vi "ReadWaveform.vi"(7 "Poll Time (ms)":u32=10, 8 "error in":errorcluster, 9 "Timeout (s)":dbl=5.0, 10 "Samps Read per Chan":i32, 11 "Task in":refnum<class "WaveformTask.lvclass">) -> (0 "error out":errorcluster, 1 "Samples Remaining":u32, 2 "Waveforms":waveform(sgl)[](array[waveform]), 3 "Task out":refnum<class "WaveformTask.lvclass">)   [LabVIEW 2015, in "WaveformTask.lvclass"]
uses:
  WaveformTask.lvclass
  WaveformTask.lvclass/WaveformTask.ctl
  <vilib>/NI/cRIO Wfm/ErrorSelector.ctl
  <vilib>/rvi/errors/niLvFpgaAdjustHostInterfaceError.vi
  <vilib>/Utility/error.llb/Error Cluster From Error Code.vi
  DataFIFOs.ctl
  <vilib>/rvi/interface/nirviMethod/nirviMethod.xnode
  <vilib>/NI/cRIO Wfm/cRIO Wfm.lvlib
  <vilib>/FPGAPlugInAG/Dynamic/niLvFpga_ReadFifo_Dynamic.vi
  <vilib>/rvi/errors/niLvFpgaMergeErrorWithErrorCode.vi
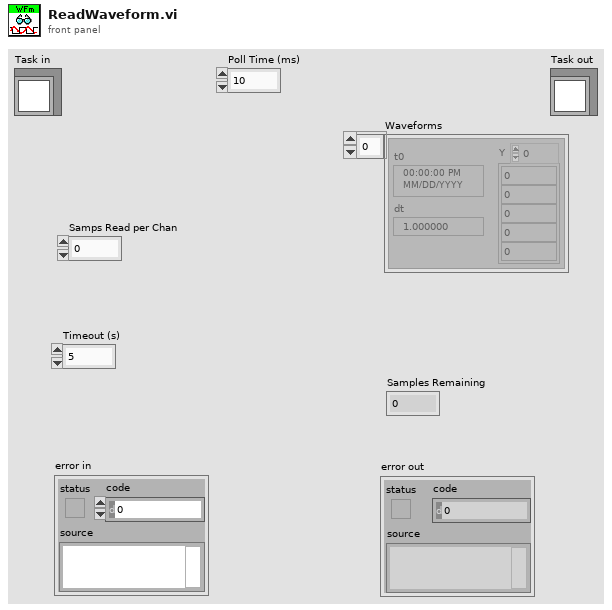
[diagram p1: front panel]
types:
  T1 = typedef "WaveformTask.lvclass/DataFIFOs.ctl" = refnum<k20>
  T2 = typedef "cRIO Wfm.lvlib/ErrorSelector.ctl" = enum16{"Read Timeout", "Module Underflow", "DMA Overflow", "Chan Count", "Run Timeout", "Start Timeout", "Stop Timeout"}
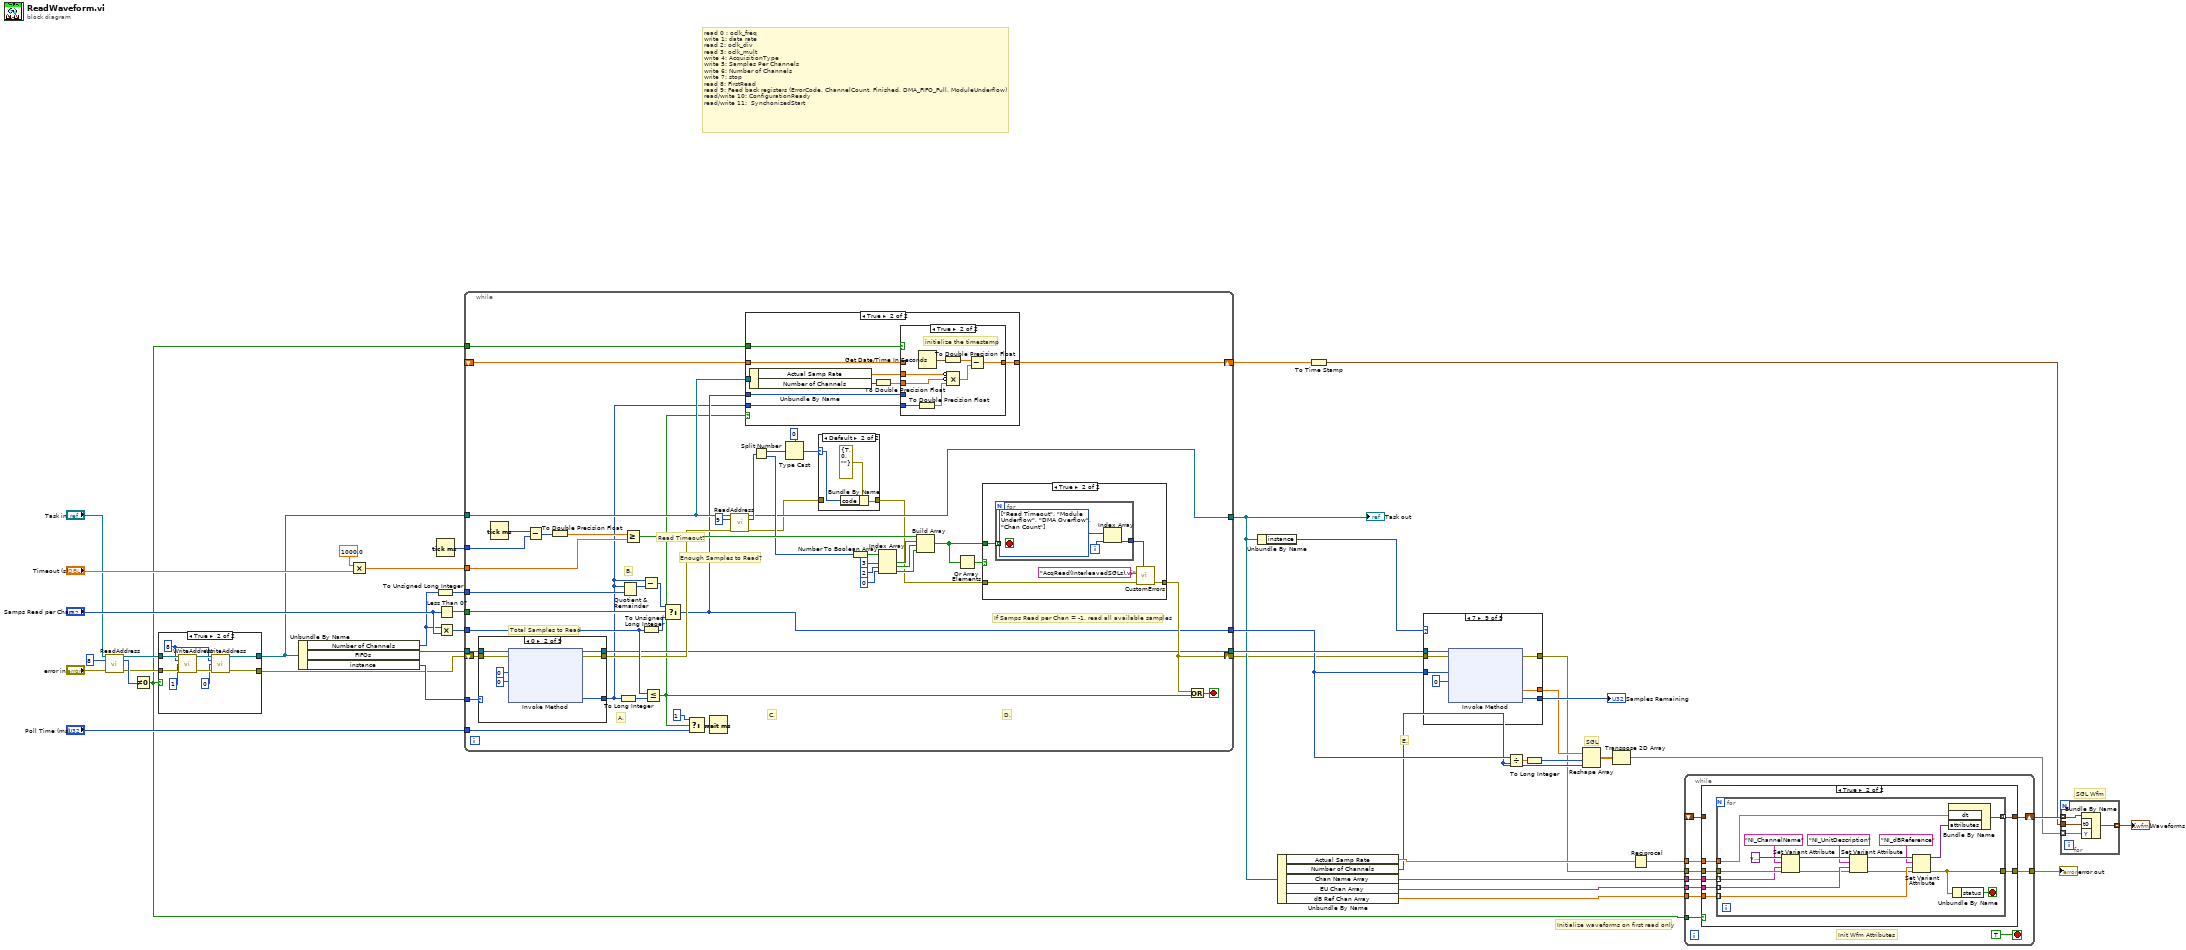
[diagram p0: block diagram]
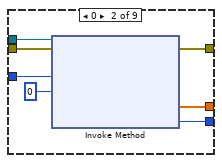
[diagram p5: hidden frame]
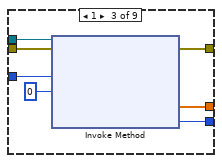
[diagram p6: hidden frame]
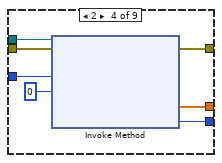
[diagram p7: hidden frame]
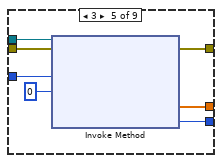
[diagram p8: hidden frame]
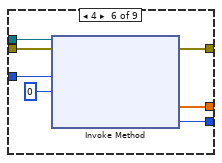
[diagram p9: hidden frame]
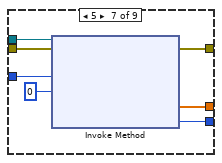
[diagram p10: hidden frame]
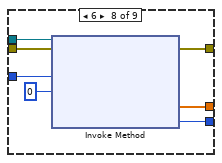
[diagram p11: hidden frame]
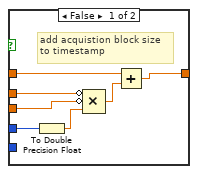
[diagram p13: hidden frame]
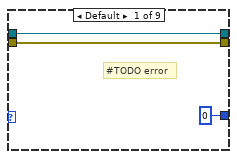
[diagram p15: hidden frame]
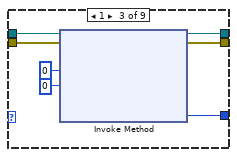
[diagram p16: hidden frame]
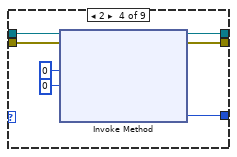
[diagram p17: hidden frame]
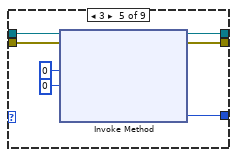
[diagram p18: hidden frame]
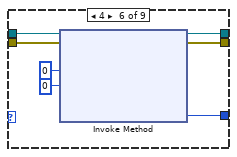
[diagram p19: hidden frame]
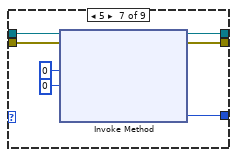
[diagram p20: hidden frame]
diagram:
  # "Initialize waveforms on first read only"
  # "SGL Wfm"
  # "SGL"
  # "read 0 : oclk_freq\nwrite 1: data rate\nread 2: oclk_div\nread 3: oclk_mult\nwrite 4: AcquisitionType\nwrite 5: Samples Per Channels\nwrite 6: Number of Channels\nwrite 7: stop\nread 8: FirstRead\nread 9: Feed back registers (ErrorCode, ChannelCount, Finished, DMA_FIFO_Full, ModuleUnderflow)\nread/write 10: ConfigurationReady\nread/write 11:  SynchonizedStart"
  # "E."
  n1 = call "ReadAddress.vi"("Task in"="Task in", "address"=u64 8, "error in (no error)"="error in") -> ("Task out"=w6:refnum<class "WaveformTask.lvclass">, "data"=w7:u64, "error out"=w5:errorcluster)  [unwired: 10 in]
  n2 = Not Equal To 0?(x=w7) -> (x != 0?=w2:bool)
  n3 = case shown="True" w2 {
    tunnel: w6 -> [w46 w55]
    tunnel: w5 -> [w45 w54]
    tunnel: [w46 w48] -> w4
    tunnel: [w45 w47] -> w3
    frame False {
    }
    frame True {
      w51 = u64 8 ("address")
      n4 = call "WriteAddress.vi"("Task in"=w55, "address"=w51, "data"=u64 1, "error in (no error)"=w54) -> ("Task out"=w53:refnum<class "WaveformTask.lvclass">, "error out"=w52:errorcluster)  [unwired: 10 in]
      n5 = call "WriteAddress.vi"("Task in"=w53, "address"=w51, "data"=u64 0, "error in (no error)"=w52) -> ("Task out"=w48:refnum<class "WaveformTask.lvclass">, "error out"=w47:errorcluster)  [unwired: 10 in]
    }
  }
  n6 = Unbundle By Name(w4) -> ("Number of Channels"=w32:i32, "FIFOs"=w33:T1, "instance"=w31:u8)
  n7 = Multiply(x=1000.0 ("y"), y="Timeout (s)") -> (x*y=w42:dbl)
  n8 = To Unsigned Long Integer(number=w32) -> (unsigned 32bit integer=w38:u32)
  n9 = Tick Count (ms)() -> (millisecond timer value=w44:u32)
  n10 = Less Than 0?(x="Samps Read per Chan") -> (x < 0?=w40:bool)
  n11 = Multiply(x=w32, y="Samps Read per Chan") -> (x*y=w39:i32)
  n12 = while {
    tunnel: [w68] -> w41
    tunnel: w33 -> [w98]
    tunnel: w44 -> [w100]
    tunnel: w42 -> [w99]
    tunnel: "Poll Time (ms)" -> [w93]
    tunnel: [w58] -> w25
    tunnel: w39 -> [w88]
    tunnel: w40 -> [w89]
    tunnel: w38 -> [w90]
    shift-right: [w82] -> w16
    shift-left: w3 -> [w97]
    tunnel: w4 -> [w62]
    tunnel: [w67] -> w18
    tunnel: w31 -> [w66]
    tunnel: w2 -> [w61]
    shift-right: [w60] -> w1
    shift-left: _ -> [w59]
    stop <- w103 stop-if-true
    # "A."
    # "D."
    # "C."
    # "B."
    # "If Samps Read per Chan = -1, read all available samples"
    # "Read Timeout?"
    # "Total Samples to Read"
    # "Enough Samples to Read?"
    n13 = case shown="0" w66 {
      tunnel: w98 -> [w135 w142 w149 w156 w163 w170 w177 w184 w191]
      tunnel: w97 -> [w134 w141 w148 w155 w162 w169 w176 w183 w190]
      tunnel: [u32 0 ("Elements Remaining") w138 w145 w152 w159 w166 w173 w180 w187] -> w56
      tunnel: [w134 w137 w144 w151 w158 w165 w172 w179 w186] -> w75
      tunnel: [w135 w136 w143 w150 w157 w164 w171 w178 w185] -> w68
      frame Default {
        # "#TODO error"
      }
      frame 0 {
        n14 = xnode "Invoke Method"("FPGA VI Reference In"=w142, "error in"=w141, "Number of Elements"=u32 0, "Timeout (ms)"=0) -> ("FPGA VI Reference Out"=w136:T1, "error out"=w137:errorcluster, "Elements Remaining"=w138:u32)  [unwired: 1 out]
      }
      frame 1 {
        n15 = xnode "Invoke Method"("FPGA VI Reference In"=w149, "error in"=w148, "Number of Elements"=u32 0, "Timeout (ms)"=0) -> ("FPGA VI Reference Out"=w143:T1, "error out"=w144:errorcluster, "Elements Remaining"=w145:u32)  [unwired: 1 out]
      }
      frame 2 {
        n16 = xnode "Invoke Method"("FPGA VI Reference In"=w156, "error in"=w155, "Number of Elements"=u32 0, "Timeout (ms)"=0) -> ("FPGA VI Reference Out"=w150:T1, "error out"=w151:errorcluster, "Elements Remaining"=w152:u32)  [unwired: 1 out]
      }
      frame 3 {
        n17 = xnode "Invoke Method"("FPGA VI Reference In"=w163, "error in"=w162, "Number of Elements"=u32 0, "Timeout (ms)"=0) -> ("FPGA VI Reference Out"=w157:T1, "error out"=w158:errorcluster, "Elements Remaining"=w159:u32)  [unwired: 1 out]
      }
      frame 4 {
        n18 = xnode "Invoke Method"("FPGA VI Reference In"=w170, "error in"=w169, "Number of Elements"=u32 0, "Timeout (ms)"=0) -> ("FPGA VI Reference Out"=w164:T1, "error out"=w165:errorcluster, "Elements Remaining"=w166:u32)  [unwired: 1 out]
      }
      frame 5 {
        n19 = xnode "Invoke Method"("FPGA VI Reference In"=w177, "error in"=w176, "Number of Elements"=u32 0, "Timeout (ms)"=0) -> ("FPGA VI Reference Out"=w171:T1, "error out"=w172:errorcluster, "Elements Remaining"=w173:u32)  [unwired: 1 out]
      }
      frame 6 {
        n20 = xnode "Invoke Method"("FPGA VI Reference In"=w184, "error in"=w183, "Number of Elements"=u32 0, "Timeout (ms)"=0) -> ("FPGA VI Reference Out"=w178:T1, "error out"=w179:errorcluster, "Elements Remaining"=w180:u32)  [unwired: 1 out]
      }
      frame 7 {
        n21 = xnode "Invoke Method"("FPGA VI Reference In"=w191, "error in"=w190, "Number of Elements"=u32 0, "Timeout (ms)"=0) -> ("FPGA VI Reference Out"=w185:T1, "error out"=w186:errorcluster, "Elements Remaining"=w187:u32)  [unwired: 1 out]
      }
    }
    n22 = Tick Count (ms)() -> (millisecond timer value=w96:u32)
    n23 = Subtract(x=w96, y=w100) -> (x-y=w102:u32)
    n24 = To Double Precision Float(number=w102) -> (double precision float=w101:dbl)
    n25 = To Long Integer(number=w56) -> (32bit integer=w91:i32)
    n26 = Quotient & Remainder(x=w56, y=w90) -> (x-y*floor(x/y)=w86:u32)  [unwired: 1 out]
    n27 = Greater Or Equal?(x=w101, y=w99) -> (x >= y?=w95:bool)
    n28 = Subtract(x=w56, y=w86) -> (x-y=w85:u32)
    n29 = To Unsigned Long Integer(number=w88) -> (unsigned 32bit integer=w87:u32)
    n30 = Less Or Equal?(x=w88, y=w91) -> (x <= y?=w57:bool)
    n31 = Select(t=w85, s=w89, f=w87) -> (s? t:f=w58:u32)
    n32 = Select(t=u32 1, s=w57, f=w93) -> (s? t:f=w94:u32)
    n33 = Wait (ms)(milliseconds to wait=w94) -> ()  [unwired: 1 out]
    n34 = call "ReadAddress.vi"("Task in"=w62, "address"=u64 9, "error in (no error)"=w75) -> ("Task out"=w67:refnum<class "WaveformTask.lvclass">, "data"=w80:u64, "error out"=w64:errorcluster)  [unwired: 10 in]
    n35 = case shown="True" w57 {
      tunnel: w59 -> [w104 w113]
      tunnel: w61 -> [_ w112]
      tunnel: w62 -> [_ w110]
      tunnel: w56 -> [_ w109]
      tunnel: [w104 w108] -> w60
      tunnel: w58 -> [_ w107]
      frame False {
      }
      frame True {
        n36 = Unbundle By Name(w110) -> ("Actual Samp Rate"=w111:dbl, "Number of Channels"=w106:i32)
        n37 = To Double Precision Float(number=w106) -> (double precision float=w105:dbl)
        n38 = case shown="True" w112 {
          tunnel: w111 -> [w118 w128]
          tunnel: w113 -> [w119 _]
          tunnel: w107 -> [w115 _]
          tunnel: w105 -> [w116 w127]
          tunnel: w109 -> [_ w122]
          tunnel: [w120 w124] -> w108
          frame False {
            # "add acquistion block size\nto timestamp"
            n39 = To Double Precision Float(number=w115) -> (double precision float=w114:dbl)
            n40 = Compound Arithmetic op=MULTIPLY(invert w118, invert w116, w114) -> (w117:dbl)
            n41 = Add(x=w119, y=w117) -> (x+y=w120:dbl)
          }
          frame True {
            # "initialize the timestamp"
            n42 = To Double Precision Float(number=w122) -> (double precision float=w121:dbl)
            n43 = Get Date/Time In Seconds() -> (seconds since 1Jan1904=w126:timestamp)
            n44 = To Double Precision Float(number=w126) -> (double precision float=w123:dbl)
            n45 = Compound Arithmetic op=MULTIPLY(invert w128, invert w127, w121) -> (w125:dbl)
            n46 = Subtract(x=w123, y=w125) -> (x-y=w124:dbl)
          }
        }
      }
    }
    n47 = Split Number(x=w80) -> (hi(x)=w79:u32, lo(x)=w77:u32)
    n48 = Type Cast(type=0, x=w79) -> (*(type *) &x=w65:i32)
    n49 = case shown="Default" w65 {
      selector: w65 -> [_ w131]
      tunnel: w64 -> [w129 _]
      tunnel: [w129 w130] -> w63
      frame 0 {
      }
      frame Default {
        n50 = Bundle By Name(cluster=errorcluster {"status"=TRUE, "code"=0, "source"=""} ("error out"), "code"=w131) -> (w130:errorcluster)
      }
    }
    n51 = Number To Boolean Array(number=w77) -> (Boolean array=w76:bool[])
    n52 = Index Array(array=w76, index #1=3 ("index"), index #2=2 ("index"), index #3=0 ("index")) -> (element #1=w71:bool, element #2=w70:bool, element #3=w69:bool)
    n53 = Build Array(w95, w71, w70, w69) -> (w83:bool[])
    n54 = Or Array Elements(Boolean array=w83) -> (logical OR=w84:bool)
    n55 = case shown="True" w84 {
      tunnel: [w192 w196] -> w82
      tunnel: w63 -> [w192 w197]
      tunnel: w83 -> [_ w195]
      frame False {
      }
      frame True {
        n56 = for {
          tunnel: w195 -> [w201] mode=indexing
          tunnel: [w198] -> w194
          i -> [w199]
          stop <- w201 stop-if-true
          w200 = T2[] [enum."Read Timeout", enum."Module Underflow", enum."DMA Overflow", enum."Chan Count"] items=["Read Timeout", "Module Underflow", "DMA Overflow", "Chan Count", "Run Timeout", "Start Timeout", "Stop Timeout"]
          n57 = Index Array(array=w200, index=w199) -> (element=w198:T2)
        }
        n58 = call <vilib>:"CustomErrors.vi"("Error Selector"=w194, "error in"=w197, "Calling VI"="AcqRead(InterleavedSGLs).vi") -> ("error out"=w196:errorcluster)  [unwired: 8 in]
      }
    }
    n59 = Or(x=w82, y=w57) -> (x .or. y?=w103:bool)
  }
  "Task out" <- w18
  n60 = Unbundle By Name(w18) -> ("instance"=w30:u8)
  n61 = Unbundle By Name(w18) -> ("Actual Samp Rate"=w24:dbl, "Number of Channels"=w17:i32, "Chan Name Array"=w20:string[], "EU Chan Array"=w21:string[], "dB Ref Chan Array"=w22:dbl[])
  n62 = To Time Stamp(1:w1) -> (0:w12:timestamp)
  n63 = case shown="7" w30 {
    tunnel: [w202 w209 w216 w223 w230 w237 w244 w251 w258] -> w15
    tunnel: w16 -> [w202 w208 w215 w222 w229 w236 w243 w250 w257]
    tunnel: w41 -> [_ w207 w214 w221 w228 w235 w242 w249 w256]
    tunnel: w25 -> [_ w206 w213 w220 w227 w234 w241 w248 w255]
    tunnel: [_ w204 w211 w218 w225 w232 w239 w246 w253] -> w26
    tunnel: [_ w203 w210 w217 w224 w231 w238 w245 w252] -> w34
    frame Default {
      # "#TODO Error"
    }
    frame 0 {
      n64 = xnode "Invoke Method"("FPGA VI Reference In"=w207, "error in"=w208, "Number of Elements"=w206, "Timeout (ms)"=0) -> ("error out"=w209:errorcluster, "Data"=w204:sgl[], "Elements Remaining"=w203:u32)  [unwired: 1 out]
    }
    frame 1 {
      n65 = xnode "Invoke Method"("FPGA VI Reference In"=w214, "error in"=w215, "Number of Elements"=w213, "Timeout (ms)"=0) -> ("error out"=w216:errorcluster, "Data"=w211:sgl[], "Elements Remaining"=w210:u32)  [unwired: 1 out]
    }
    frame 2 {
      n66 = xnode "Invoke Method"("FPGA VI Reference In"=w221, "error in"=w222, "Number of Elements"=w220, "Timeout (ms)"=0) -> ("error out"=w223:errorcluster, "Data"=w218:sgl[], "Elements Remaining"=w217:u32)  [unwired: 1 out]
    }
    frame 3 {
      n67 = xnode "Invoke Method"("FPGA VI Reference In"=w228, "error in"=w229, "Number of Elements"=w227, "Timeout (ms)"=0) -> ("error out"=w230:errorcluster, "Data"=w225:sgl[], "Elements Remaining"=w224:u32)  [unwired: 1 out]
    }
    frame 4 {
      n68 = xnode "Invoke Method"("FPGA VI Reference In"=w235, "error in"=w236, "Number of Elements"=w234, "Timeout (ms)"=0) -> ("error out"=w237:errorcluster, "Data"=w232:sgl[], "Elements Remaining"=w231:u32)  [unwired: 1 out]
    }
    frame 5 {
      n69 = xnode "Invoke Method"("FPGA VI Reference In"=w242, "error in"=w243, "Number of Elements"=w241, "Timeout (ms)"=0) -> ("error out"=w244:errorcluster, "Data"=w239:sgl[], "Elements Remaining"=w238:u32)  [unwired: 1 out]
    }
    frame 6 {
      n70 = xnode "Invoke Method"("FPGA VI Reference In"=w249, "error in"=w250, "Number of Elements"=w248, "Timeout (ms)"=0) -> ("error out"=w251:errorcluster, "Data"=w246:sgl[], "Elements Remaining"=w245:u32)  [unwired: 1 out]
    }
    frame 7 {
      n71 = xnode "Invoke Method"("FPGA VI Reference In"=w256, "error in"=w257, "Number of Elements"=w255, "Timeout (ms)"=0) -> ("error out"=w258:errorcluster, "Data"=w253:sgl[], "Elements Remaining"=w252:u32)  [unwired: 1 out]
    }
  }
  "Samples Remaining" <- w34
  n72 = Divide(x=w25, y=w17) -> (x/y=w28:dbl)
  n73 = To Long Integer(number=w28) -> (32bit integer=w27:i32)
  n74 = Reshape Array(w26, w27, w17) -> (w29:sgl[][])
  n75 = Transpose 2D Array(2D array=w29) -> (transposed array=w14:sgl[][])
  n76 = Reciprocal(x=w24) -> (1/x=w23:dbl)
  n77 = while {
    tunnel: w23 -> [w268]
    tunnel: w22 -> [w267]
    tunnel: w15 -> [w266]
    tunnel: [w265] -> w13
    tunnel: w21 -> [w264]
    tunnel: w20 -> [w263]
    shift-right: [w262] -> w19
    shift-left: _ -> [w260]
    tunnel: w2 -> [w259]
    stop <- TRUE stop-if-true
    # "Init Wfm Attributes"
    n78 = case shown="True" w259 {
      tunnel: w268 -> [_ w277]
      tunnel: w267 -> [_ w276]
      tunnel: w266 -> [w270 w275]
      tunnel: [w270 w274] -> w265
      tunnel: w264 -> [_ w273]
      tunnel: w263 -> [_ w272]
      tunnel: [w269 w271] -> w262
      tunnel: w260 -> [w269 _]
      frame False {
      }
      frame True {
        n79 = for {
          tunnel: w277 -> [w294]
          tunnel: [w293] -> w271 mode=indexing
          tunnel: w273 -> [w291] mode=indexing
          tunnel: w276 -> [w287] mode=indexing
          tunnel: w275 -> [w290]
          tunnel: [w289] -> w274
          tunnel: w272 -> [w278] mode=indexing
          stop <- w288 stop-if-true
          n80 = Set Variant Attribute(Variant=variant ("variant out"), name="NI_ChannelName", value=w278, error in=w290) -> (Variant out=w283:variant, error out=w285:errorcluster)  [unwired: 1 out]
          n81 = Set Variant Attribute(Variant=w283, name="NI_UnitDescription", value=w291, error in=w285) -> (Variant out=w284:variant, error out=w286:errorcluster)  [unwired: 1 out]
          n82 = Set Variant Attribute(Variant=w284, name="NI_dBReference", value=w287, error in=w286) -> (Variant out=w292:variant, error out=w289:errorcluster)  [unwired: 1 out]
          n83 = Bundle By Name("dt"=w294, "attributes"=w292) -> (w293:waveform(sgl))  [unwired: 1 out]
          n84 = Unbundle By Name(w289) -> ("status"=w288:bool)
        }
      }
    }
  }
  "error out" <- w13
  n85 = for {
    tunnel: w19 -> [w298] mode=indexing
    tunnel: w12 -> [w297]
    tunnel: [w296] -> w11 mode=indexing
    tunnel: w14 -> [w295] mode=indexing
    n86 = Bundle By Name(cluster=w298, "t0"=w297, "Y"=w295) -> (w296:waveform(sgl))
  }
  "Waveforms" <- w11
